vi "SetMotors_ReadEncoders_SubVI.vi"() -> ()   [LabVIEW 2018]
panel:
  in  "PID gains":T1(array[cluster])=[{"proportional gain (Kc)"=1.0, "integral time (Ti, min)"=0.01, "derivative time (Td, min)"=0.0}] {"derivative time (Td, min)" format="%.3f"; "integral time (Ti, min)" format="%.3f"; "proportional gain (Kc)" format="%.3f"}
  in  "steering frame velocity":dbl[](array[numeric])=[0.0, 0.0, 0.0]
  out "ccw motor velocity setpoints":dbl[](array[numeric])
  out "Radians/s":dbl[](array[numeric])
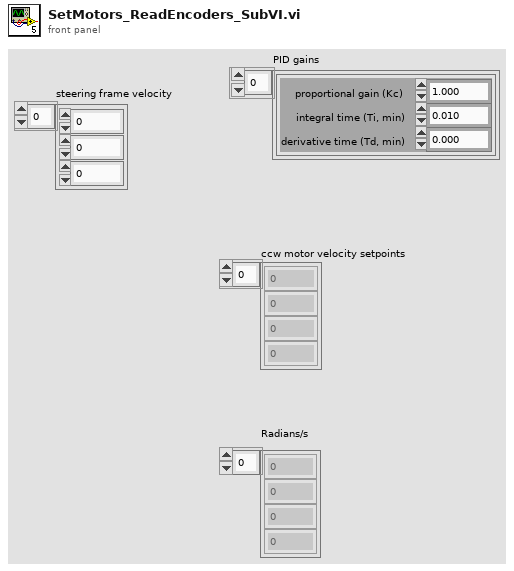
[diagram p1: front panel]
types:
  T1 = cluster{"proportional gain (Kc)":dbl, "integral time (Ti, min)":dbl, "derivative time (Td, min)":dbl}[]
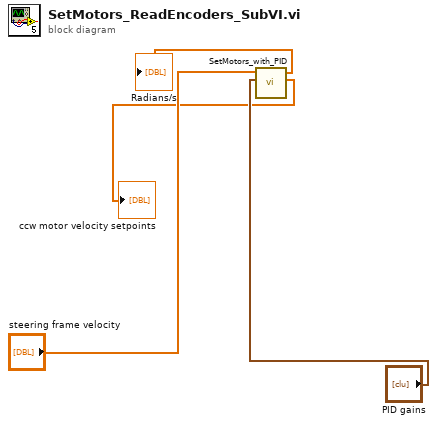
[diagram p0: block diagram]
diagram:
  n1 = call "SetMotors_with_PID.vi"("PID gains"="PID gains", "steering frame velocity"="steering frame velocity") -> ("ccw motor velocity setpoints"=→"ccw motor velocity setpoints":dbl[], "Radians/s"=→"Radians/s":dbl[])  [unwired: 8 in]
